vi "ReceiveSendMessageResponse.vi"(8 "error in (no error)":errorcluster, 11 "body":variant) -> (0 "error out":errorcluster, 1 "error code":i32, 3 "message":T1, 4 "error info":string)   [LabVIEW 2017, in "ServerComm.lvlib"]
doc: "Returns response \nmessages from services in reply to messages that the device sent them."
uses:
  <vilib>/addons/InsightCM/Devices/Shared/Common/ServerComm/ServerComm.lvlib
  <vilib>/addons/InsightCM/MessageBus/Base/controls/Message.ctl
  <vilib>/addons/InsightCM/MessageBus/Base/controls/MessageHeader.ctl
  <vilib>/addons/InsightCM/MessageBus/Base/controls/KeyValuePair.ctl
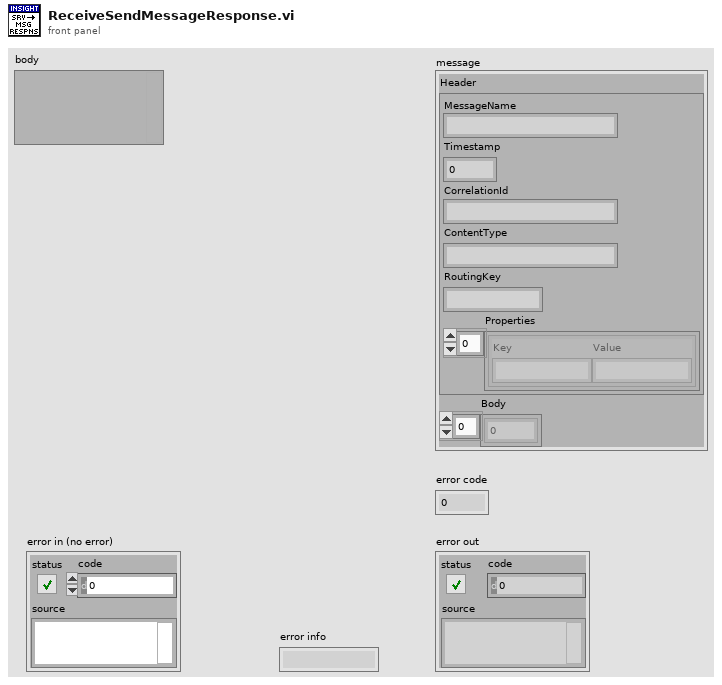
[diagram p1: front panel]
types:
  T1 = typedef "Message.ctl" = cluster{"Header":T2, "Body":u8[]}
  T2 = typedef "MessageHeader.ctl" = cluster{"MessageName":string, "Timestamp":i64, "CorrelationId":string, "ContentType":string, "RoutingKey":string, "Properties":T3[]}
  T3 = typedef "KeyValuePair.ctl" = cluster{"Key":string, "Value":string}
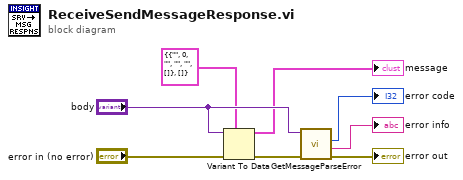
[diagram p0: block diagram]
diagram:
  n1 = Variant To Data(error in="error in (no error)", type=T1 {"Header"={"MessageName"="", "Timestamp"=0, "CorrelationId"="", "ContentType"="", "RoutingKey"="", "Properties"=[]}, "Body"=[]} ("Message"), Variant="body") -> (data=→"message":T1, error out=w7:errorcluster)
  n2 = call <vilib>:"GetMessageParseError.vi"("error in (no error)"=w7, "body"="body") -> ("error out"=→"error out":errorcluster, "error info"=→"error info":string, "error code"=→"error code":i32)  [unwired: 7 in]
